vi "Control Panel.vi"(8 "error in (no error)":errorcluster, 11 "TC in":refnum<class "Temperature Controller.lvclass">) -> (0 "error out":errorcluster, 3 "TC out":refnum<class "Temperature Controller.lvclass">)   [LabVIEW 2009, in "Temperature Controller.lvclass"]
uses:
  Temperature Controller.lvclass
  AutoCtl.ctl
  HV Slide Indicator.ctl
  Utility Classes/InstrPtr/InstrPtr.lvclass
  Global/Relative Sound Files.vi
  Temperature Controller.lvclass/Temperature Controller.ctl
  File IO/File IO.lvclass
  Utility Classes/Readable/Readable.lvclass
panel:
  in  "SET":bool
  in  "New Temp":dbl[unit]
  in  "Update interval":dbl[unit]=0.5 min=0.1 max=10.0
  out "*itc503":T1
  out "Currently":dbl[unit]
  in  "Stable Sensitivity +-":dbl=0.05 caption="+/-" min=0.0 step=0.1
  out "stable":bool caption="Stable"
  in  "Set Point":dbl[unit]=6.0 min=0.0 max=305.0
  out "Internal refresh event signal":bool
  in  "Warn At":dbl[unit]
  in  "Comparison":bool
  in  "Alarm?":bool caption="Boolean"
  in  "Time to Fill":dbl[unit]
  in  "Fill VTI":bool
  out "Time Remaining":string caption="Time"
  in  "Timer?":bool
  out "done?":bool
  in  "clear":bool
  out "Timer start time":timestamp
  in  "Display":dbl[unit]=600.0
  in  "autoscale?":bool=TRUE
  out "Temperature graph":T2(graph)
  out "active":bool
  out "Auto Indicator":T3={"Auto Heater"=FALSE, "Auto Needle"=FALSE, "Auto PID"=TRUE}
  in  "Auto Controls":T4={"Heater"=FALSE, "Needle"=FALSE, "PID"=TRUE}
  out "Ndisbar":T5 caption="Needle Valve              (est. %)" max=100.0 scale=0.0..100.0 scale format="%.1f"
  in  "Ncontrol":dbl(slide) min=0.0 max=100.0 scale=0.0..100.0
  in  "Hcontrol":dbl(slide) min=0.0 max=99.9 scale=0.0..100.0
  out "Hdispbar":T5 caption="Heater" max=100.0 scale=0.0..100.0 scale format="%.1f"
  out "ready?":bool
  in  "Check for TC":bool
  in  "endprgm":bool
  # "Temperature Controller"
  # "Greater"
  # "Less"
  # "Manual"
  # "Auto"
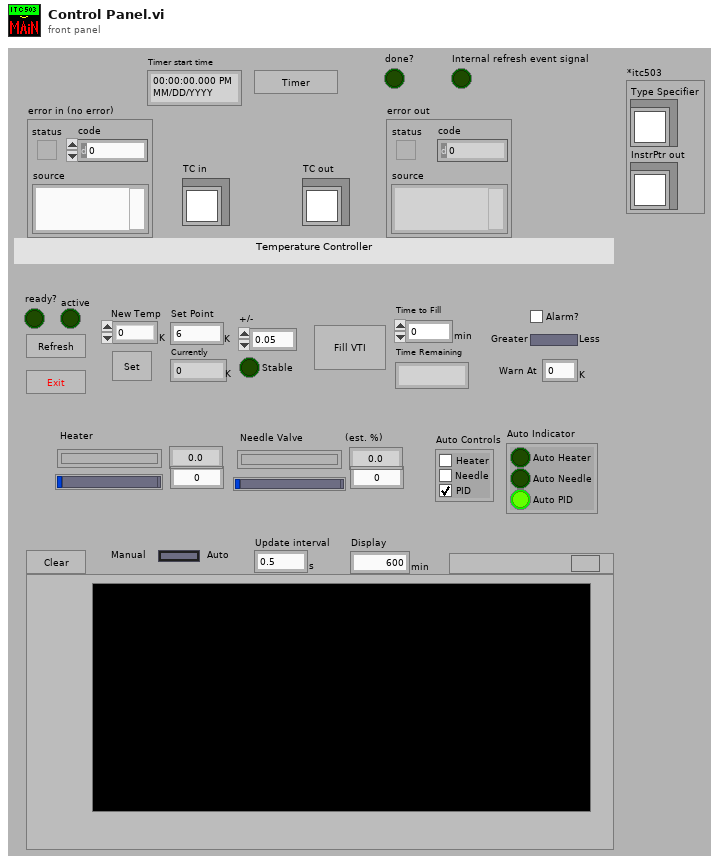
[diagram p1: front panel]
types:
  T1 = cluster{"Type Specifier":refnum<class "Temperature Controller.lvclass">, "InstrPtr out":refnum<class "InstrPtr.lvclass">}
  T2 = cluster{"Data Points":cluster{"t":timestamp, "x":dbl}[]}[]
  T3 = typedef "Temperature Controller.lvclass/AutoCtl.ctl" = cluster{"Auto Heater":bool, "Auto Needle":bool, "Auto PID":bool}
  T4 = cluster{"Heater":bool, "Needle":bool, "PID":bool}
  T5 = typedef "Temperature Controller.lvclass/HV Slide Indicator.ctl" = dbl
  T6 = enum8{"Enabled", "Disabled", "Disabled and Grayed Out"}
  T7 = cluster{"Type Specifier":refnum<class "Temperature Controller.lvclass">, "Instrument Pointer":refnum<class "InstrPtr.lvclass">}
  T8 = typedef "Readable.lvclass/TX Graph.ctl" = cluster{"Data Points":cluster{"t":timestamp, "x":dbl}[]}[]
  T9 = cluster{"Data Points":cluster{"t":timestamp, "x":dbl}[]}
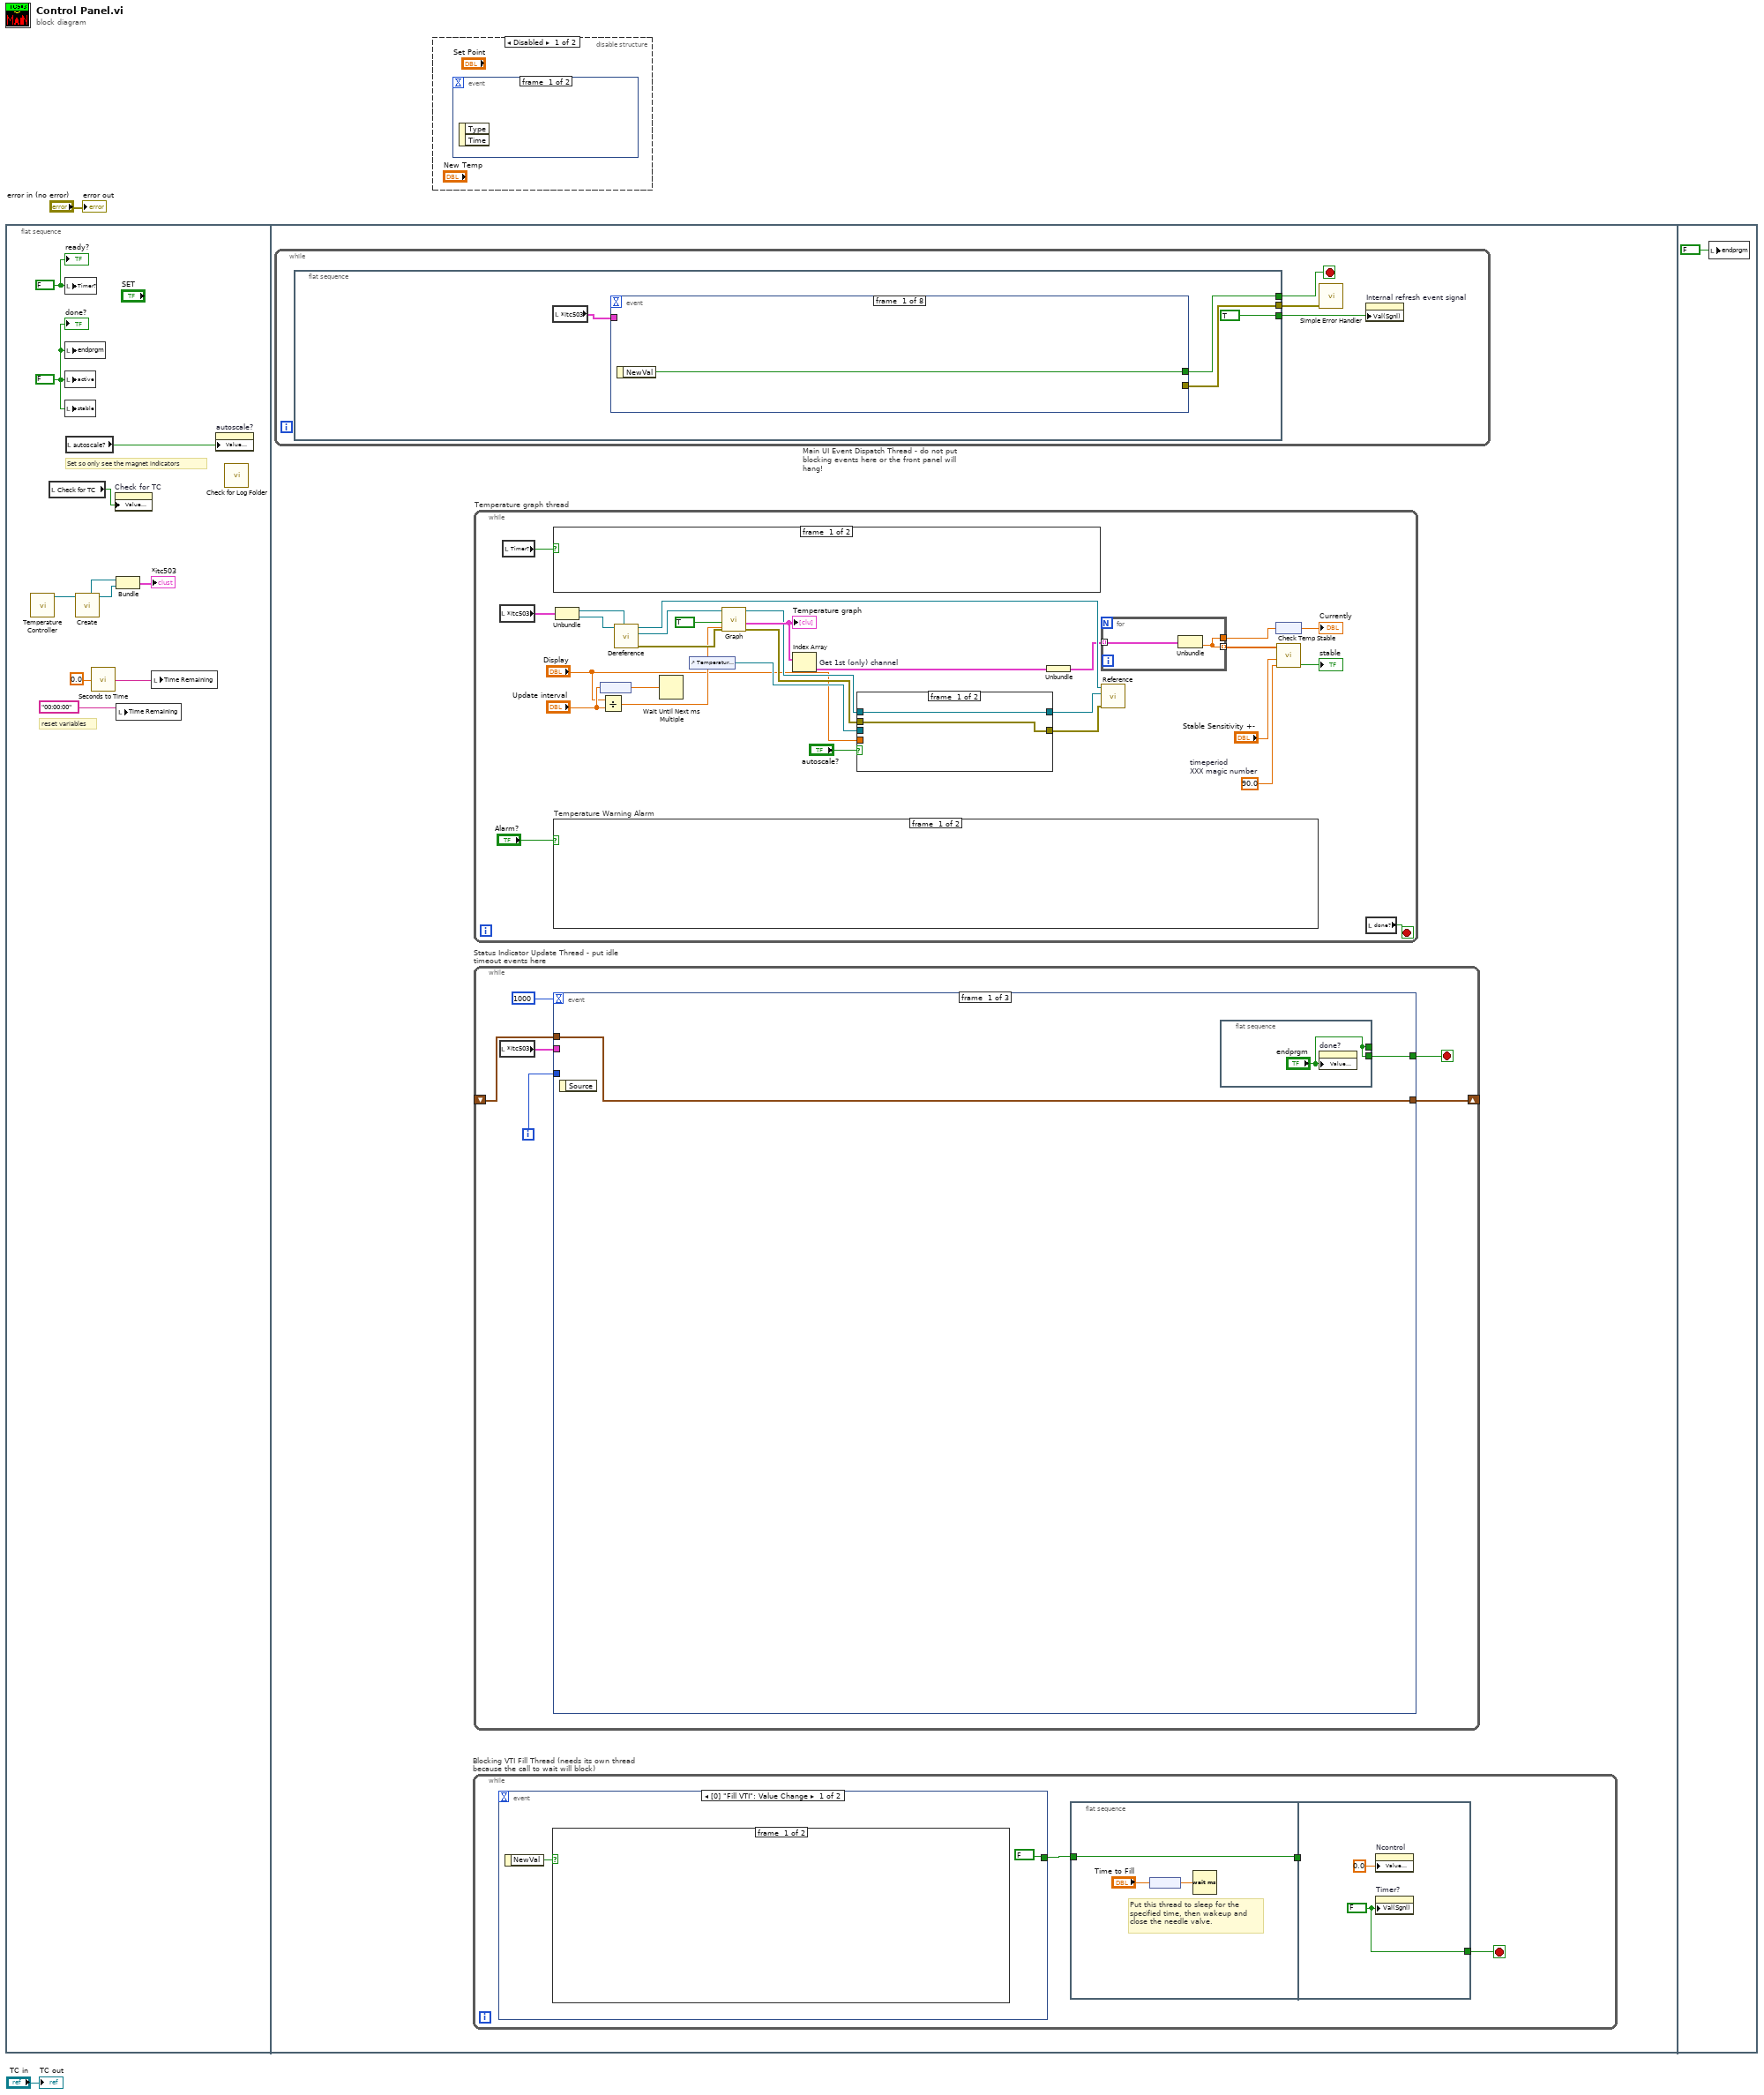
[diagram p0: block diagram]
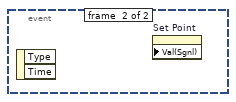
[diagram p2: hidden frame]
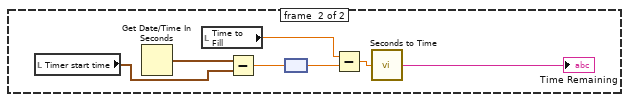
[diagram p4: hidden frame]
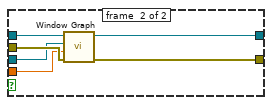
[diagram p5: hidden frame]
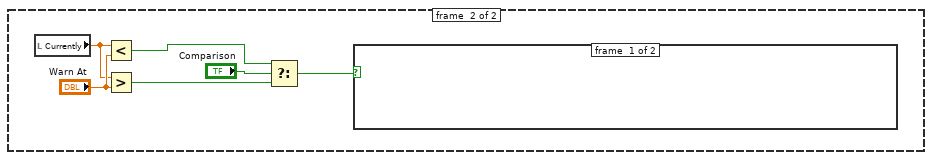
[diagram p6: hidden frame]
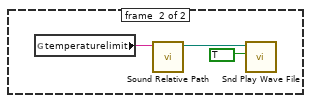
[diagram p7: hidden frame]
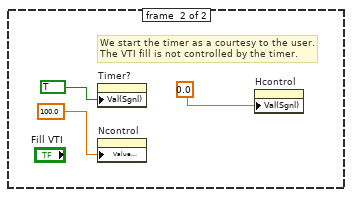
[diagram p8: hidden frame]
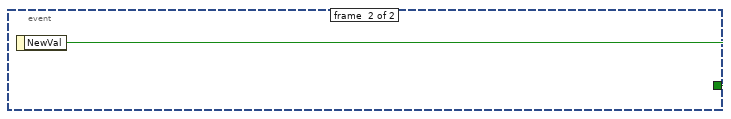
[diagram p9: hidden frame]
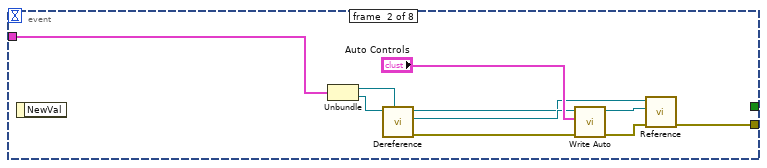
[diagram p10: hidden frame]
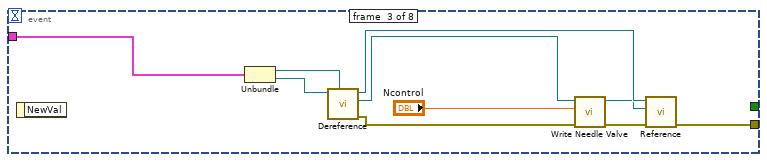
[diagram p11: hidden frame]
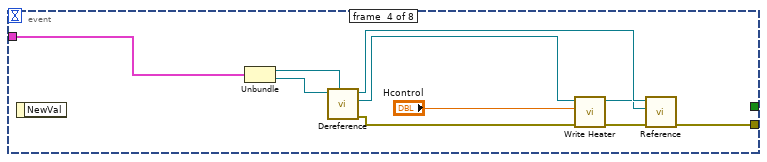
[diagram p12: hidden frame]
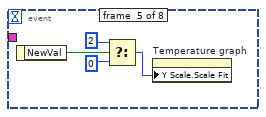
[diagram p13: hidden frame]
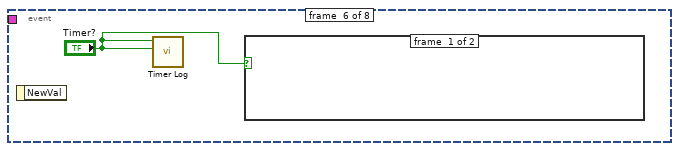
[diagram p14: hidden frame]
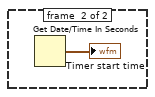
[diagram p15: hidden frame]
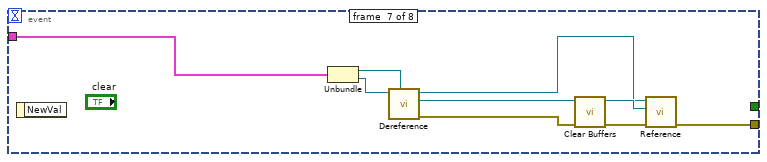
[diagram p16: hidden frame]
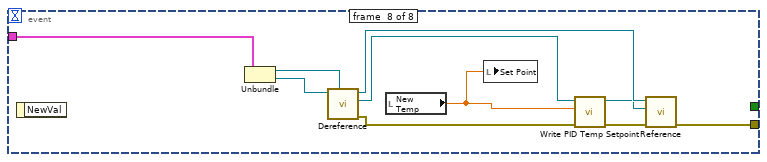
[diagram p17: hidden frame]
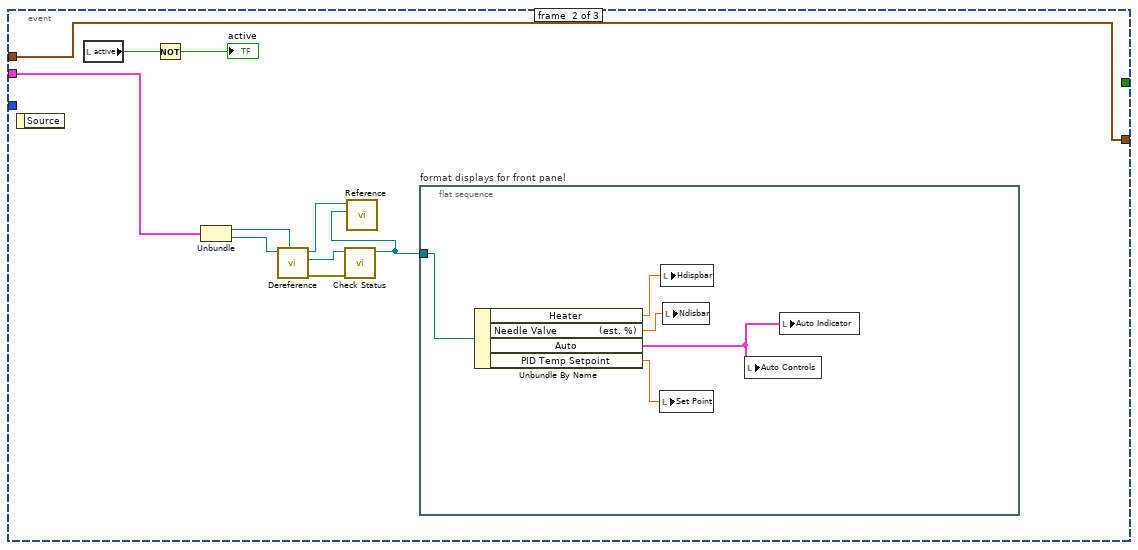
[diagram p18: hidden frame]
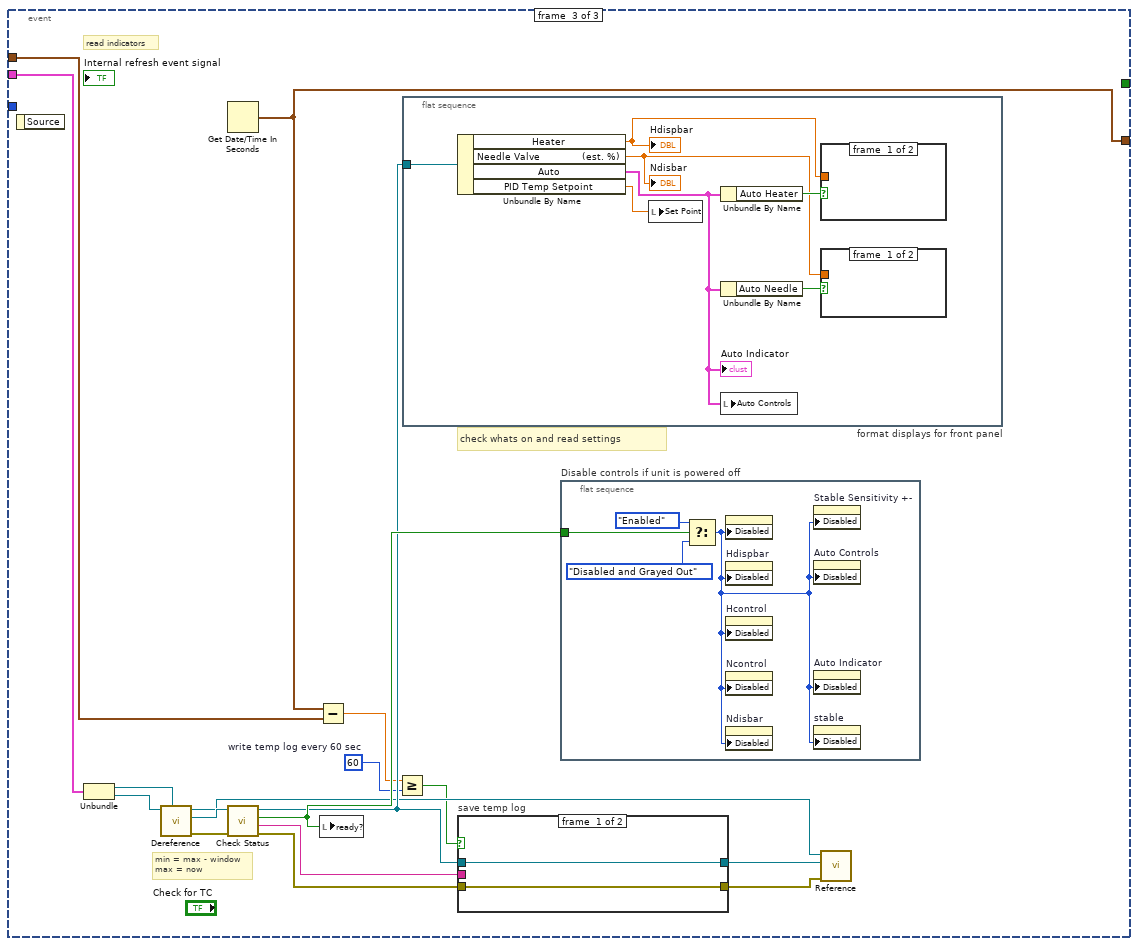
[diagram p19: hidden frame]
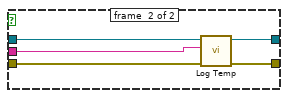
[diagram p20: hidden frame]
diagram:
  n1 = flat-sequence {
    frame #0 {
      w13 = FALSE
      w9 = FALSE
      # "Set so only see the magnet indicators"
      # "reset variables"
      n2 = call "Temperature Controller.vi"() -> ("Temperature Controller out"=w8:refnum<class "Temperature Controller.lvclass">)  [unwired: 10 in, 1 out]
      n3 = local read "Check for TC"() -> (w10:bool)
      n4 = local write "Timer?"(w13) -> ()
      n5 = local write "endprgm"(w9) -> ()
      n6 = local write "active"(w9) -> ()
      n7 = local write "stable"(w9) -> ()
      n8 = local read "autoscale?"() -> (w11:bool)
      n9 = call "Create.vi"("Instrument in"=w8) -> ("Instrument Pointer"=w6:refnum<class "InstrPtr.lvclass">, "Type Specifier"=w7:refnum<class "Temperature Controller.lvclass">)  [unwired: 8 in, 1 out]
      n10 = call "Seconds to Time.vi"("Seconds"=dbl[unit] 0.0) -> ("Time"=w4:string)
      n11 = property on="Check for TC" class="Bool (strict)"("Value (Signaling)"=w10) -> ()  [unwired: 2 in, 2 out]
      n12 = Bundle("Type Specifier"=w7, "Instrument Pointer"=w6) -> (→"*itc503":T7)  [unwired: 1 in]
      n13 = local write "Time Remaining"("00:00:00") -> ()
      n14 = local write "Time Remaining"(w4) -> ()
      n15 = property on="autoscale?" class="Boolean (strict)"("Value (Signaling)"=w11) -> ()  [unwired: 2 in, 2 out]
      n16 = call "Check for Log Folder.vi"() -> ()  [unwired: 1 out]
      "ready?" <- w13
      "done?" <- w9
    }
    frame #1 {
      n17 = while "Main UI Event Dispatch Thread - do not put blocking events here or the front panel will hang!" {
        stop <- w85 stop-if-true
        n18 = flat-sequence {
          tunnel: [w89] -> w84
          tunnel: [w88] -> w85
          tunnel: [TRUE ("Value (Signaling)")] -> w83
          frame #0 {
            n19 = local read "*itc503"() -> (w87:T1)
            n20 = event shown="[7] \"Set Point\", \"SET\": Value Change" {
              selector: _ -> [_ _ _ _ _ _ _ _]
              dyn-events: _ -> [_ _ _ _ _ _ _ _]
              timeout: _ -> [_ _ _ _ _ _ _ _]
              tunnel: [w90 _ _ _ _ _ _ _] -> w88
              tunnel: w87 -> [_ w96 w106 w116 _ _ w130 w142]
              tunnel: [_ w97 w107 w117 _ _ w127 w143] -> w89
              event #0 {
                n21 = event-data() -> ("NewVal"=w90:bool)  [unwired: 1 out]
              }
              event #1 {
                n22 = event-data() -> ()  [unwired: 2 out]
                n23 = Unbundle(w96) -> ("Type Specifier"=w92:refnum<class "Temperature Controller.lvclass">, "InstrPtr out"=w91:refnum<class "InstrPtr.lvclass">)
                n24 = call "Dereference.vi"("Type Specifier"=w92, "InstrPtr"=w91) -> ("error out"=w99:errorcluster, "Instrument out"=w95:refnum<class "Temperature Controller.lvclass">, "InstrPtr out"=w94:refnum<class "InstrPtr.lvclass">)  [unwired: 7 in]
                n25 = call-dynamic "Write Auto.vi"("error in (no error)"=w99, "Auto"="Auto Controls", "Temperature Controller in"=w95) -> ("error out"=w98:errorcluster, "Temperature Controller out"=w93:refnum<class "Temperature Controller.lvclass">)  [unwired: 7 in]
                n26 = call "Reference.vi"("error in (no error)"=w98, "Instrument"=w93, "InstrPtr in"=w94) -> ("error out"=w97:errorcluster)  [unwired: 8 in]
              }
              event #2 {
                n27 = event-data() -> ()  [unwired: 2 out]
                n28 = Unbundle(w106) -> ("Type Specifier"=w102:refnum<class "Temperature Controller.lvclass">, "InstrPtr out"=w101:refnum<class "InstrPtr.lvclass">)
                n29 = call "Dereference.vi"("Type Specifier"=w102, "InstrPtr"=w101) -> ("error out"=w108:errorcluster, "Instrument out"=w105:refnum<class "Temperature Controller.lvclass">, "InstrPtr out"=w104:refnum<class "InstrPtr.lvclass">)  [unwired: 7 in]
                n30 = call-dynamic "Write Needle Valve.vi"("error in (no error)"=w108, "Heater"="Ncontrol", "Temperature Controller in"=w105) -> ("error out"=w109:errorcluster, "Temperature Controller out"=w103:refnum<class "Temperature Controller.lvclass">)  [unwired: 7 in]
                n31 = call "Reference.vi"("error in (no error)"=w109, "Instrument"=w103, "InstrPtr in"=w104) -> ("error out"=w107:errorcluster)  [unwired: 8 in]
              }
              event #3 {
                n32 = event-data() -> ()  [unwired: 2 out]
                n33 = Unbundle(w116) -> ("Type Specifier"=w111:refnum<class "Temperature Controller.lvclass">, "InstrPtr out"=w112:refnum<class "InstrPtr.lvclass">)
                n34 = call "Dereference.vi"("Type Specifier"=w111, "InstrPtr"=w112) -> ("error out"=w119:errorcluster, "Instrument out"=w115:refnum<class "Temperature Controller.lvclass">, "InstrPtr out"=w114:refnum<class "InstrPtr.lvclass">)  [unwired: 7 in]
                n35 = call-dynamic "Write Heater.vi"("error in (no error)"=w119, "Heater"="Hcontrol", "Temperature Controller in"=w115) -> ("error out"=w118:errorcluster, "Temperature Controller out"=w113:refnum<class "Temperature Controller.lvclass">)  [unwired: 7 in]
                n36 = call "Reference.vi"("error in (no error)"=w118, "Instrument"=w113, "InstrPtr in"=w114) -> ("error out"=w117:errorcluster)  [unwired: 8 in]
              }
              event #4 {
                n37 = event-data() -> ("NewVal"=w121:bool)  [unwired: 1 out]
                n38 = Select(t=2, s=w121, f=0) -> (s? t:f=w124:i32)
                n39 = property on="Temperature graph" class="XYGraph (strict)"("Y Scale.Scale Fit"=w124) -> ()  [unwired: 2 in, 2 out]
              }
              event #5 {
                n40 = event-data() -> ()  [unwired: 2 out]
                n41 = call "Timer Log.vi"("flag"="Timer?", "toggle"="Timer?") -> ()  [unwired: 10 out]
                n42 = case shown="True" "Timer?" {
                  frame #0 {
                  }
                  frame #1 {
                    n43 = Get Date/Time In Seconds() -> (seconds since 1Jan1904=→"Timer start time":timestamp)
                  }
                }
              }
              event #6 {
                n44 = event-data() -> ()  [unwired: 2 out]
                n45 = Unbundle(w130) -> ("Type Specifier"=w131:refnum<class "Temperature Controller.lvclass">, "InstrPtr out"=w132:refnum<class "InstrPtr.lvclass">)
                n46 = call "Dereference.vi"("Type Specifier"=w131, "InstrPtr"=w132) -> ("error out"=w129:errorcluster, "Instrument out"=w135:refnum<class "Temperature Controller.lvclass">, "InstrPtr out"=w133:refnum<class "InstrPtr.lvclass">)  [unwired: 7 in]
                n47 = call "Clear Buffers.vi"("error in (no error)"=w129, "Readable in"=w135) -> ("error out"=w128:errorcluster, "Readable out"=w134:refnum<class "Temperature Controller.lvclass">)  [unwired: 8 in]
                n48 = call "Reference.vi"("error in (no error)"=w128, "Instrument"=w134, "InstrPtr in"=w133) -> ("error out"=w127:errorcluster)  [unwired: 8 in]
              }
              event #7 {
                n49 = event-data() -> ()  [unwired: 2 out]
                n50 = Unbundle(w142) -> ("Type Specifier"=w138:refnum<class "Temperature Controller.lvclass">, "InstrPtr out"=w137:refnum<class "InstrPtr.lvclass">)
                n51 = call "Dereference.vi"("Type Specifier"=w138, "InstrPtr"=w137) -> ("error out"=w144:errorcluster, "Instrument out"=w140:refnum<class "Temperature Controller.lvclass">, "InstrPtr out"=w141:refnum<class "InstrPtr.lvclass">)  [unwired: 7 in]
                n52 = local read "New Temp"() -> (w136:dbl[unit])
                n53 = local write "Set Point"(w136) -> ()
                n54 = call-dynamic "Write PID Temp Setpoint.vi"("error in (no error)"=w144, "PID Temp Setpoint"=w136, "Temperature Controller in"=w140) -> ("error out"=w145:errorcluster, "Temperature Controller out"=w139:refnum<class "Temperature Controller.lvclass">)  [unwired: 7 in]
                n55 = call "Reference.vi"("error in (no error)"=w145, "Instrument"=w139, "InstrPtr in"=w141) -> ("error out"=w143:errorcluster)  [unwired: 8 in]
              }
            }
          }
        }
        n56 = call <vilib>:"Simple Error Handler.vi"("error in (no error)"=w84) -> ()  [unwired: 4 in, 5 out]
        n57 = property on="Internal refresh event signal" class="Bool (strict)"("Val(Sgnl)"=w83) -> ()  [unwired: 2 in, 2 out]
      }
      n58 = while "Blocking VTI Fill Thread (needs its own thread because the call to wait will block)" {
        stop <- w69 stop-if-true
        n59 = event shown="[0] \"Fill VTI\": Value Change" {
          selector: _ -> [_ _]
          dyn-events: _ -> [_ _]
          timeout: _ -> [_ _]
          tunnel: [FALSE ("NewVal") w82] -> w70
          event #0 {
            n60 = event-data() -> ("NewVal"=w77:bool)  [unwired: 1 out]
            n61 = case shown="True" w77 {
              frame #0 {
              }
              frame #1 {
                # "We start the timer as a courtesy to the user.\nThe VTI fill is not controlled by the timer."
                n62 = property on="Timer?" class="Bool (strict)"("Val(Sgnl)"=TRUE ("Value (Signaling)")) -> ()  [unwired: 2 in, 2 out]
                n63 = property on="Ncontrol" class="Slide (strict)"("Value (Signaling)"=100.0 ("Ncontrol")) -> ()  [unwired: 2 in, 2 out]
                n64 = property on="Hcontrol" class="Slide (strict)"("Val(Sgnl)"=0.0 ("Ncontrol")) -> ()  [unwired: 2 in, 2 out]
              }
            }
          }
          event #1 {
            n65 = event-data() -> ("NewVal"=w82:bool)  [unwired: 1 out]
          }
        }
        n66 = flat-sequence {
          tunnel: [w72] -> w71
          tunnel: w70 -> [w72]
          tunnel: w71 -> [_]
          tunnel: [w75] -> w69
          frame #0 {
            # "Put this thread to sleep for the specified time, then wakeup and close the needle valve."
            n67 = node("Time to Fill") -> (w73:dbl)
            n68 = Wait (ms)(milliseconds to wait=w73) -> ()  [unwired: 1 out]
          }
          frame #1 {
            w75 = FALSE ("Value (Signaling)")
            n69 = property on="Ncontrol" class="Slide (strict)"("Value (Signaling)"=0.0 ("Ncontrol")) -> ()  [unwired: 2 in, 2 out]
            n70 = property on="Timer?" class="Bool (strict)"("Val(Sgnl)"=w75) -> ()  [unwired: 2 in, 2 out]
          }
        }
      }
      n71 = while "Temperature graph thread" {
        stop <- w23 stop-if-true
        w35 = 90.0  # timeperiod XXX magic number
        n72 = local read "*itc503"() -> (w31:T1)
        n73 = local read "Timer?"() -> (w24:bool)
        n74 = case shown="True" w24 {
          frame #0 {
          }
          frame #1 {
            n75 = local read "Timer start time"() -> (w48:timestamp)
            n76 = Get Date/Time In Seconds ("jkl;jkljkl")() -> (seconds since 1Jan1904=w49:timestamp)
            n77 = local read "Time to Fill"() -> (w45:dbl[unit])
            n78 = Subtract(x=w49, y=w48) -> (x-y=w51:dbl)
            n79 = node(w51) -> (w47:dbl[unit])
            n80 = Subtract(x=w45, y=w47) -> (x-y=w46:dbl[unit])
            n81 = call "Seconds to Time.vi"("Seconds"=w46) -> ("Time"=→"Time Remaining":string)
          }
        }
        n82 = case "Temperature Warning Alarm" shown="True" "Alarm?" {
          frame #0 {
          }
          frame #1 {
            n83 = local read "Currently"() -> (w60:dbl[unit])
            n84 = Less?(x=w60, y="Warn At") -> (x < y?=w64:bool)
            n85 = Greater?(x=w60, y="Warn At") -> (0:w63:bool)
            n86 = Select(t=w64, s="Comparison", f=w63) -> (s? t:f=w62:bool)
            n87 = case shown="True" w62 {
              frame #0 {
              }
              frame #1 {
                n88 = global read "Relative Sound Files.vi" "temperaturelimit"() -> (w67:string)
                n89 = call "Sound Relative Path.vi"("Sound"=w67) -> ("Relative Path"=w66:path)  [unwired: 10 in]
                n90 = call <vilib>:"Snd Play Wave File.vi"("wait until finish (T)"=TRUE, "wave file path"=w66) -> ()  [unwired: 1 in, 9 out]
              }
            }
          }
        }
        n91 = Unbundle(w31) -> ("Type Specifier"=w36:refnum<class "Temperature Controller.lvclass">, "InstrPtr out"=w37:refnum<class "InstrPtr.lvclass">)
        n92 = node("Update interval") -> (w22:dbl)
        n93 = Divide(x="Display", y="Update interval") -> (x/y=w20:dbl)
        n94 = call "Dereference.vi"("Type Specifier"=w36, "InstrPtr"=w37) -> ("error out"=w40:errorcluster, "Instrument out"=w39:refnum<class "Temperature Controller.lvclass">, "InstrPtr out"=w38:refnum<class "InstrPtr.lvclass">)  [unwired: 7 in]
        n95 = Wait Until Next ms Multiple(millisecond multiple=w22) -> ()  [unwired: 1 out]
        n96 = control-ref of="Temperature graph"() -> (w15:refnum<vi>)
        n97 = call-dynamic "Graph.vi"("Ring size (points) (1024)"=w20, "error in (no error)"=w40, "Store Ring? (f)"=TRUE, "Readable in"=w39) -> ("error out"=w19:errorcluster, "Ring Buffers"=w30:T8, "Readable out"=w18:refnum<class "Temperature Controller.lvclass">)  [unwired: 1 in, 4 out]
        "Temperature graph" <- w30
        n98 = Index Array "Get 1st (only) channel"(array=w30) -> (element=w29:T9)  [unwired: 1 in]
        n99 = case shown="True" "autoscale?" {
          tunnel: w19 -> [w52 w59]
          tunnel: w18 -> [w53 w58]
          tunnel: [w53 w57] -> w17
          tunnel: [w52 w56] -> w16
          tunnel: w15 -> [_ w55]
          tunnel: "Display" -> [_ w54]
          frame #0 {
          }
          frame #1 {
            n100 = call-dynamic "Window Graph.vi"("error in (no error)"=w59, "Window"=w54, "Graph ref"=w55, "Readable in"=w58) -> ("error out"=w56:errorcluster, "Readable out"=w57:refnum<class "Temperature Controller.lvclass">)  [unwired: 6 in]
          }
        }
        n101 = Unbundle(w29) -> ("Data Points"=w28:cluster{"t":timestamp, "x":dbl}[])
        n102 = for {
          tunnel: w28 -> [w44] mode=indexing
          tunnel: [w43] -> w27 mode=indexing
          tunnel: [w43] -> w26
          n103 = Unbundle(w44) -> ("x"=w43:dbl)  [unwired: 1 out]
        }
        n104 = call "Reference.vi"("error in (no error)"=w16, "Instrument"=w17, "InstrPtr in"=w38) -> ()  [unwired: 8 in, 1 out]
        n105 = node(w26) -> (→"Currently":dbl[unit])
        n106 = call "Check Temp Stable.vi"("timeperiod"=w35, "sens"="Stable Sensitivity +-", "temparray"=w27) -> ("stable"=→"stable":bool)  [unwired: 8 in]
        n107 = local read "done?"() -> (w23:bool)
      }
      n108 = while "Status Indicator Update Thread - put idle timeout events here" {
        shift-right: [w147] -> _
        shift-left: _ -> [w148]
        i -> [w149]
        stop <- w150 stop-if-true
        n109 = local read "*itc503"() -> (w146:T1)
        n110 = event shown="[2] \"Check for TC\", \"Internal refresh event signal\": Value Change" {
          selector: _ -> [_ _ _]
          dyn-events: _ -> [_ _ _]
          timeout: 1000 -> [_ _ _]
          tunnel: [w152 _ _] -> w150
          tunnel: w149 -> [_ _ _]
          tunnel: w148 -> [w153 w162 w184]
          tunnel: [w153 w162 w186] -> w147
          tunnel: w146 -> [_ w161 w185]
          event #0 {
            n111 = event-data() -> ()  [unwired: 2 out]
            n112 = flat-sequence {
              tunnel: ["endprgm"] -> _
              tunnel: ["endprgm"] -> w152
              frame #0 {
                n113 = property on="done?" class="Boolean (strict)"("Value (Signaling)"="endprgm") -> ()  [unwired: 2 in, 2 out]
              }
            }
          }
          event #1 {
            n114 = event-data() -> ()  [unwired: 2 out]
            n115 = local read "active"() -> (w164:bool)
            n116 = Not(x=w164) -> (.not. x?=→"active":bool)
            n117 = Unbundle(w161) -> ("Type Specifier"=w157:refnum<class "Temperature Controller.lvclass">, "InstrPtr out"=w158:refnum<class "InstrPtr.lvclass">)
            n118 = call "Dereference.vi"("Type Specifier"=w157, "InstrPtr"=w158) -> ("error out"=w160:errorcluster, "Instrument out"=w159:refnum<class "Temperature Controller.lvclass">, "InstrPtr out"=w156:refnum<class "InstrPtr.lvclass">)  [unwired: 7 in]
            n119 = call-dynamic "Check Status.vi"("error in (no error)"=w160, "Temperature Controller in"=w159) -> ("Temperature Controller out"=w155:refnum<class "Temperature Controller.lvclass">)  [unwired: 6 in, 3 out]
            n120 = call "Reference.vi"("Instrument"=w155, "InstrPtr in"=w156) -> ()  [unwired: 9 in, 1 out]
            n121 = flat-sequence "format displays for front panel" {
              tunnel: w155 -> [w169]
              frame #0 {
                n122 = Unbundle By Name(w169) -> ("Heater"=w166:T5, "Needle Valve              (est. %)"=w167:T5, "Auto"=w165:T3, "PID Temp Setpoint"=w168:dbl[unit])
                n123 = local write "Set Point"(w168) -> ()
                n124 = local write "Hdispbar"(w166) -> ()
                n125 = local write "Ndisbar"(w167) -> ()
                n126 = local write "Auto Controls"(w165) -> ()
                n127 = local write "Auto Indicator"(w165) -> ()
              }
            }
          }
          event #2 {
            w174 = 60  # write temp log every 60 sec
            # "min = max - window\nmax = now"
            # "read indicators"
            # "check whats on and read settings"
            n128 = event-data() -> ()  [unwired: 2 out]
            n129 = Unbundle(w185) -> ("Type Specifier"=w182:refnum<class "Temperature Controller.lvclass">, "InstrPtr out"=w181:refnum<class "InstrPtr.lvclass">)
            n130 = call "Dereference.vi"("Type Specifier"=w182, "InstrPtr"=w181) -> ("error out"=w176:errorcluster, "Instrument out"=w180:refnum<class "Temperature Controller.lvclass">, "InstrPtr out"=w177:refnum<class "InstrPtr.lvclass">)  [unwired: 7 in]
            n131 = Get Date/Time In Seconds() -> (seconds since 1Jan1904=w186:timestamp)
            n132 = call-dynamic "Check Status.vi"("error in (no error)"=w176, "Temperature Controller in"=w180) -> ("error out"=w172:errorcluster, "Status"=w170:string, "Ready?"=w183:bool, "Temperature Controller out"=w179:refnum<class "Temperature Controller.lvclass">)  [unwired: 6 in]
            n133 = Subtract(x=w186, y=w184) -> (x-y=w175:dbl)
            n134 = local write "ready?"(w183) -> ()
            n135 = Greater Or Equal?(x=w175, y=w174) -> (x >= y?=w173:bool)
            n136 = flat-sequence "format displays for front panel" {
              tunnel: w179 -> [w199]
              frame #0 {
                n137 = Unbundle By Name(w199) -> ("Heater"=w203:T5, "Needle Valve              (est. %)"=w200:T5, "Auto"=w202:T3, "PID Temp Setpoint"=w198:dbl[unit])
                "Auto Indicator" <- w202
                "Ndisbar" <- w200
                "Hdispbar" <- w203
                n138 = local write "Set Point"(w198) -> ()
                n139 = Unbundle By Name(w202) -> ("Auto Heater"=w204:bool)
                n140 = Unbundle By Name(w202) -> ("Auto Needle"=w201:bool)
                n141 = local write "Auto Controls"(w202) -> ()
                n142 = case shown="True" w204 {
                  tunnel: w203 -> [_ w206]
                  frame #0 {
                  }
                  frame #1 {
                    n143 = local write "Hcontrol"(w206) -> ()
                  }
                }
                n144 = case shown="True" w201 {
                  tunnel: w200 -> [_ w205]
                  frame #0 {
                  }
                  frame #1 {
                    n145 = local write "Ncontrol"(w205) -> ()
                  }
                }
              }
            }
            n146 = case "save temp log" shown="True" w173 {
              tunnel: w179 -> [w188 w193]
              tunnel: [w188 w192] -> w178
              tunnel: w172 -> [w187 w191]
              tunnel: [w187 w190] -> w171
              tunnel: w170 -> [_ w189]
              frame #0 {
              }
              frame #1 {
                n147 = call-dynamic "Log Temp.vi"("error in (no error)"=w191, "Status string"=w189, "Temperature Controller in"=w193) -> ("error out"=w190:errorcluster, "Temperature Controller out"=w192:refnum<class "Temperature Controller.lvclass">)  [unwired: 7 in]
              }
            }
            n148 = flat-sequence "Disable controls if unit is powered off" {
              tunnel: w183 -> [w196]
              frame #0 {
                n149 = Select(t=T6."Enabled" ("Disabled"), s=w196, f=T6."Disabled and Grayed Out" ("Disabled")) -> (s? t:f=w197:T6)
                n150 = property on="Set Point" class="DigNum (strict)"("Disabled"=w197) -> ()  [unwired: 2 in, 2 out]
                n151 = property on="Hdispbar" class="Slide (strict)"("Disabled"=w197) -> ()  [unwired: 2 in, 2 out]
                n152 = property on="Hcontrol" class="Slide (strict)"("Disabled"=w197) -> ()  [unwired: 2 in, 2 out]
                n153 = property on="Ncontrol" class="Slide (strict)"("Disabled"=w197) -> ()  [unwired: 2 in, 2 out]
                n154 = property on="Ndisbar" class="Slide (strict)"("Disabled"=w197) -> ()  [unwired: 2 in, 2 out]
                n155 = property on="Stable Sensitivity +-" class="Digital (strict)"("Disabled"=w197) -> ()  [unwired: 2 in, 2 out]
                n156 = property on="Auto Controls" class="Clust (strict)"("Disabled"=w197) -> ()  [unwired: 2 in, 2 out]
                n157 = property on="Auto Indicator" class="Clust (strict)"("Disabled"=w197) -> ()  [unwired: 2 in, 2 out]
                n158 = property on="stable" class="Boolean (strict)"("Disabled"=w197) -> ()  [unwired: 2 in, 2 out]
              }
            }
            n159 = call "Reference.vi"("error in (no error)"=w171, "Instrument"=w178, "InstrPtr in"=w177) -> ()  [unwired: 8 in, 1 out]
          }
        }
      }
    }
    frame #2 {
      n160 = local write "endprgm"(FALSE) -> ()
    }
  }
  n161 = disable-structure shown="Disabled" {
    frame #0 {
      n162 = event shown="[1] \"SET\": Value Change" {
        selector: _ -> [_ _]
        dyn-events: _ -> [_ _]
        timeout: _ -> [_ _]
        event #0 {
          n163 = event-data() -> ()  [unwired: 1 in, 2 out]
        }
        event #1 {
          n164 = event-data() -> ()  [unwired: 1 in, 2 out]
          n165 = property on="Set Point" class="DigNum (strict)" props=["Val(Sgnl)"]() -> ()  [unwired: 3 in, 2 out]
        }
      }
    }
    frame #1 {
    }
  }
  "error out" <- "error in (no error)"
  "TC out" <- "TC in"
